vi "Untitled-1SubVI (1).vi"(4 "Boolean":bool, 6 "Boolean 2":bool, 7 "shuffled array":i32[][](array[numeric]), 9 "Numeric":dbl, 10 "Numeric 2":dbl, 11 "Array in":u16[][](array[numeric])) -> (2 "true":bool, 3 "Array out":u16[][](array[numeric]))   [LabVIEW 2020]
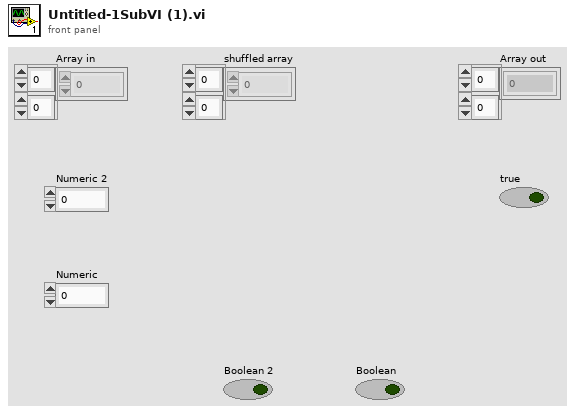
[diagram p1: front panel]
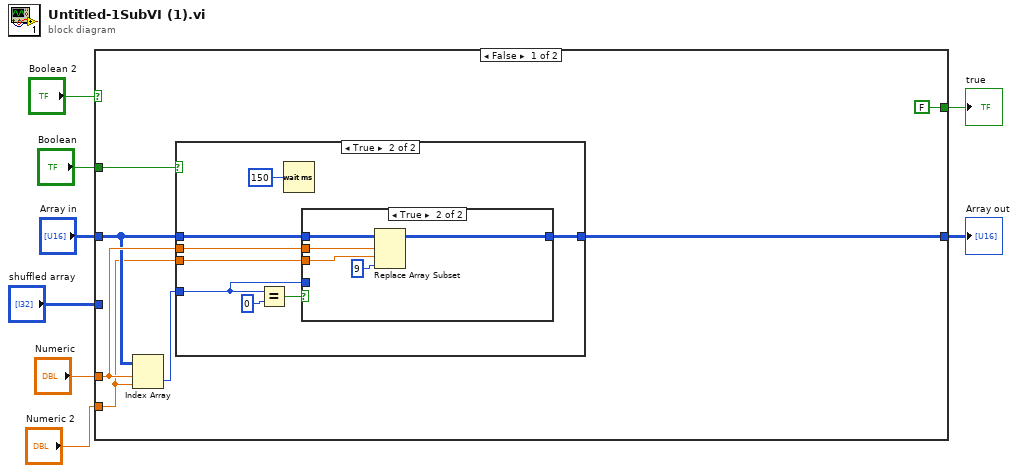
[diagram p0: block diagram]
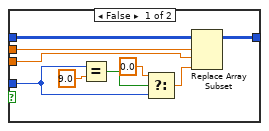
[diagram p3: hidden frame]
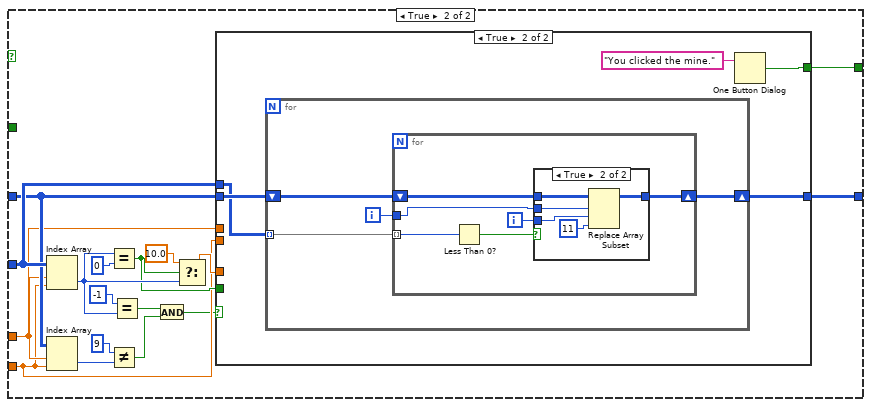
[diagram p4: hidden frame]
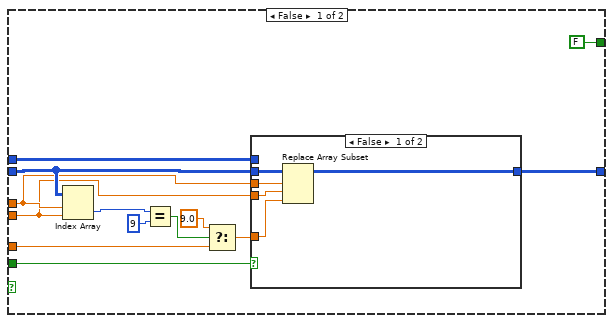
[diagram p5: hidden frame]
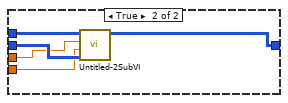
[diagram p6: hidden frame]
diagram:
  n1 = case shown="False" "Boolean 2" {
    tunnel: "Numeric 2" -> [w11 w44]
    tunnel: "Numeric" -> [w13 w45]
    tunnel: "Array in" -> [w12 w46]
    tunnel: "shuffled array" -> [_ w49]
    tunnel: [w14 w50] -> w8
    tunnel: [FALSE ("true") w54] -> w4
    tunnel: "Boolean" -> [w10 _]
    frame False {
      n2 = Index Array(array=w12, index (row)=w13, index (col)=w11) -> (element=w9:u16)
      n3 = case shown="True" w10 {
        tunnel: w12 -> [w16 w24]
        tunnel: w13 -> [_ w23]
        tunnel: w11 -> [_ w22]
        tunnel: [w16 w21] -> w14
        tunnel: w9 -> [_ w18]
        frame False {
        }
        frame True {
          n4 = Equal?(x=w18, y=u16 0) -> (x = y?=w20:bool)
          n5 = Wait (ms)(milliseconds to wait=u32 150) -> ()  [unwired: 1 out]
          n6 = case shown="True" w20 {
            tunnel: w24 -> [w29 w38]
            tunnel: w23 -> [w28 w37]
            tunnel: w22 -> [w27 w36]
            tunnel: [w25 w35] -> w21
            tunnel: w18 -> [w30 _]
            frame False {
              n7 = Equal?(x=w30, y=9.0) -> (x = y?=w32:bool)
              n8 = Select(t=0.0, s=w32, f=w30) -> (s? t:f=w26:dbl)
              n9 = Replace Array Subset(array=w29, new element=w26, index (row)=w28, index (col)=w27) -> (w25:u16[][])
            }
            frame True {
              n10 = Replace Array Subset(array=w38, new element=u16 9 ("new element/subarray"), index (row)=w37, index (col)=w36) -> (w35:u16[][])
            }
          }
        }
      }
    }
    frame True {
      n11 = Index Array(array=w49, index (row)=w45, index (col)=w44) -> (element=w51:i32)
      n12 = Index Array(array=w46, index (row)=w45, index (col)=w44) -> (element=w43:u16)
      n13 = Equal?(x=w51, y=0) -> (x = y?=w48:bool)
      n14 = Not Equal?(x=u16 9, y=w43) -> (x != y?=w41:bool)
      n15 = Equal?(x=-1, y=w51) -> (x = y?=w40:bool)
      n16 = And(x=w40, y=w41) -> (x .and. y?=w39:bool)
      n17 = Select(t=10.0, s=w48, f=w51) -> (s? t:f=w47:dbl)
      n18 = case shown="True" w39 {
        tunnel: [FALSE ("true") w82] -> w54
        tunnel: w46 -> [w64 w80]
        tunnel: w47 -> [w58 _]
        tunnel: w45 -> [w63 _]
        tunnel: w44 -> [w62 _]
        tunnel: [w67 w81] -> w50
        tunnel: w49 -> [w65 w79]
        tunnel: w48 -> [w66 _]
        frame False {
          n19 = Index Array(array=w64, index (row)=w63, index (col)=w62) -> (element=w61:u16)
          n20 = Equal?(x=w61, y=u16 9) -> (x = y?=w59:bool)
          n21 = Select(t=9.0, s=w59, f=w58) -> (s? t:f=w56:dbl)
          n22 = case shown="False" w66 {
            tunnel: w64 -> [w70 w77]
            tunnel: w56 -> [w69 _]
            tunnel: w63 -> [w72 w76]
            tunnel: w62 -> [w71 w75]
            tunnel: [w73 w74] -> w67
            tunnel: w65 -> [_ w78]
            frame False {
              n23 = Replace Array Subset(array=w70, new element=w69, index (row)=w72, index (col)=w71) -> (w73:u16[][])
            }
            frame True {
              n24 = call "Untitled-2SubVI.vi"("Array in"=w77, "Numeric 2"=w75, "Numeric"=w76, "shuffled array"=w78) -> ("Array out"=w74:u16[][])  [unwired: 7 in]
            }
          }
        }
        frame True {
          n25 = for {
            tunnel: w79 -> [w87] mode=indexing
            shift-right: [w85] -> w81
            shift-left: w80 -> [w86]
            i -> [w84]
            n26 = for {
              tunnel: w87 -> [w88] mode=indexing
              shift-right: [w91] -> w85
              shift-left: w86 -> [w92]
              tunnel: w84 -> [w90]
              i -> [w89]
              n27 = Less Than 0?(x=w88) -> (x < 0?=w93:bool)
              n28 = case shown="True" w93 {
                tunnel: w92 -> [w94 w99]
                tunnel: [w94 w98] -> w91
                tunnel: w90 -> [_ w97]
                tunnel: w89 -> [_ w96]
                frame False {
                }
                frame True {
                  n29 = Replace Array Subset(array=w99, new element=u16 11 ("new element/subarray"), index (row)=w97, index (col)=w96) -> (w98:u16[][])
                }
              }
            }
          }
          n30 = One Button Dialog(message="You clicked the mine.") -> (true=w82:bool)  [unwired: 1 in]
        }
      }
    }
  }
  "Array out" <- w8
  "true" <- w4
